vi "U64.vi"(8 "error in (no error)":errorcluster, 10 "Timeout":i32, 11 "Notifier in":refnum<class "Notifier.lvclass">) -> (0 "error out":errorcluster, 1 "Timeout?":bool, 2 "Notification Out":u64=18446744073709551615 format="%.0x", 3 "Notifier out":refnum<class "Notifier.lvclass">)   [LabVIEW 2024]
uses:
  Notifier.lvclass
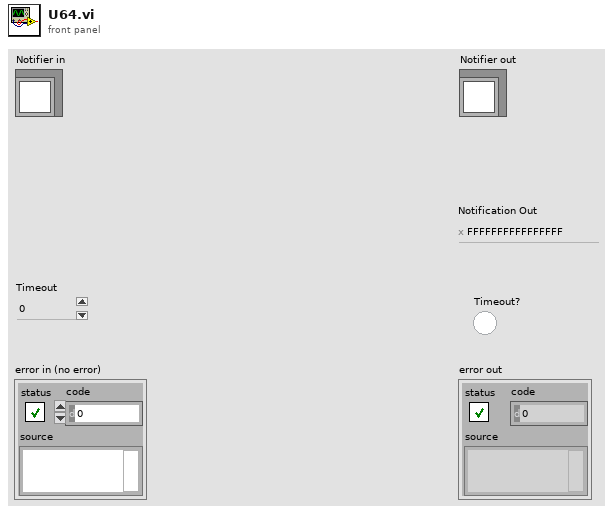
[diagram p1: front panel]
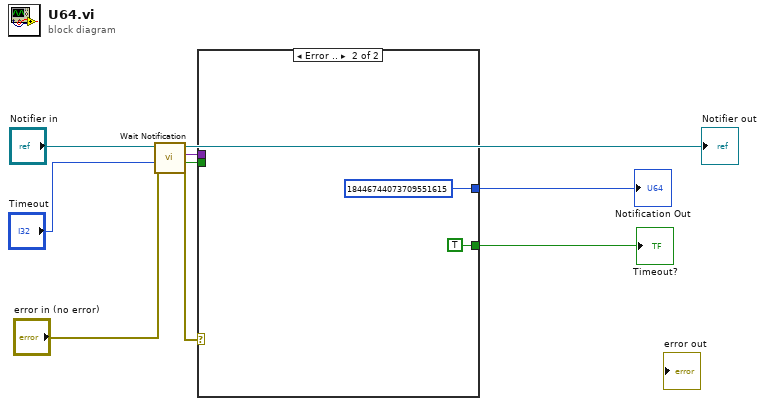
[diagram p0: block diagram]
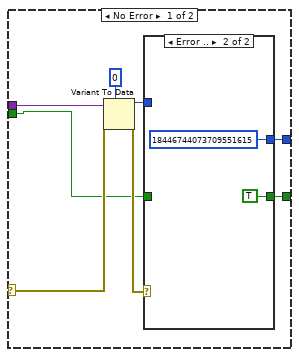
[diagram p2: hidden frame]
diagram:
  n1 = call-dynamic "Wait Notification.vi"("error in (no error)"="error in (no error)", "Timeout"="Timeout", "Notifier in"="Notifier in") -> ("error out"=w6:errorcluster, "Timeout?"=w5:bool, "Notification"=w4:variant, "Notifier out"=→"Notifier out":refnum<class "Notifier.lvclass">)  [unwired: 5 in]
  n2 = case shown="Error .." w6 {
    selector: w6 -> [w15 _]
    tunnel: w5 -> [w12 _]
    tunnel: w4 -> [w17 _]
    tunnel: [w11 TRUE ("Timeout?")] -> w2
    tunnel: [w10 u64 18446744073709551615] -> w1
    frame No Error {
      n3 = Variant To Data(error in=w15, type=u64 0, Variant=w17) -> (data=w13:u64, error out=w14:errorcluster)
      n4 = case shown="Error .." w14 {
        tunnel: w12 -> [w19 _]
        tunnel: [w19 TRUE ("Timeout?")] -> w11
        tunnel: w13 -> [w18 _]
        tunnel: [w18 u64 18446744073709551615] -> w10
        frame No Error {
        }
        frame Error {
        }
      }
    }
    frame Error {
    }
  }
  "Timeout?" <- w2
  "Notification Out" <- w1
